vi "5-1_PushCounter.vi"() -> ()   [LabVIEW 2014]
doc: "This example demonstrates how to read one channel of digital input from a LINX device.\n------------------------------------\nAuther: Koji Ohashi\nCopyright (c) 2020 Japan LabVIEW Users Group, Volunteer members.\nThis VI is released under the MIT License.\nhttp://opensource.org/licenses/mit-license.php\n------------------------------------"
uses:
  <vilib>/MakerHub/LINX/LMH-LINX.lvlib
  <vilib>/MakerHub/LINX/Public/Peripherals/Digital/Digital Read 1 Chan.vi
  <vilib>/MakerHub/LINX/Public/Utilities/Open Serial.vi
panel:
  out "Count":i32
  out "DI Value":bool
  in  "DI Channel":u8=2
  in  "Stop Button":bool
  in  "Serial Port":refnum<visa-resource-name>
  # "LINX Device Settings"
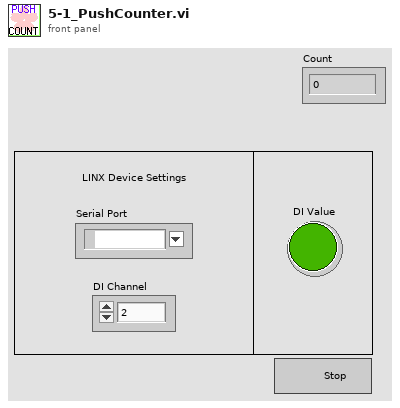
[diagram p1: front panel]
types:
  T1 = typedef "LMH-LINX.lvlib/LINX Ref.ctl" = cluster{"IO":T2, "Interface":T3, "LINX Device Config":T4}
  T2 = typedef "LMH-LINX.lvlib/Platform.ctl" = enum16{"Remote", "Local"}
  T3 = typedef "LMH-LINX.lvlib/Interface.ctl" = enum16{"Serial", "TCP"}
  T4 = typedef "LMH-LINX.lvlib/Device.lvlib/LINX Device Config.ctl" = cluster{"Interface":T3, "COM Port":refnum<visa-resource-name>, "TCP Configuration":T5, "Device Family":u8, "Device ID":u8, "Device Name":string, "TCP Ref":refnum<k5>, "Channels":T6}
  T5 = typedef "LMH-LINX.lvlib/Device.lvlib/TCP Config.ctl" = cluster{"IP Address":string, "Port":u16}
  T6 = typedef "LMH-LINX.lvlib/Channels.ctl" = cluster{"DI":u8[], "DO":u8[], "AI":u8[], "AO":u8[], "PWM":u8[], "QE":u8[], "UART":u8[], "I2C 2":u8[], "SPI":u8[], "CAN":u8[], "Servo":u8[], "AI Ref (V)":dbl, "AI Resolution (Bits)":u8, "AO Ref (V)":dbl, "AO Resolution (Bits)":u8}
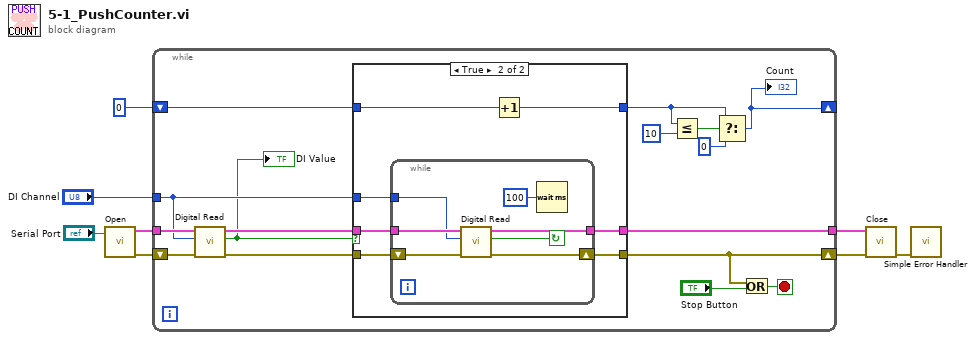
[diagram p0: block diagram]
diagram:
  n1 = call-poly <vilib>:"Open.vi"("Serial Port"="Serial Port") -> ("Error Out"=w7:errorcluster, "LINX Resource"=w8:T1)  [unwired: 8 in, 1 out]
  n2 = while {
    tunnel: w8 -> [w22]
    tunnel: [w10] -> w6
    shift-right: [w13] -> w5
    shift-left: w7 -> [w21]
    tunnel: "DI Channel" -> [w15]
    shift-right: [w17] -> _
    shift-left: 0 -> [w12]
    stop <- w24 stop-if-true
    n3 = call-poly <vilib>:"Digital Read.vi"("Error In"=w21, "DI Channel"=w15, "LINX Resource"=w22) -> ("Error Out"=w14:errorcluster, "DI Value"=w9:bool, "LINX Resource"=w16:T1)  [unwired: 6 in]
    "DI Value" <- w9
    n4 = case shown="TRUE" w9 {
      tunnel: w16 -> [w25 w34]
      tunnel: w15 -> [_ w33]
      tunnel: w14 -> [w27 w32]
      tunnel: [w27 w31] -> w13
      tunnel: w12 -> [w26 w28]
      tunnel: [w26 w30] -> w11
      tunnel: [w25 w29] -> w10
      frame False {
      }
      frame True {
        n5 = while {
          tunnel: w34 -> [w41]
          tunnel: w33 -> [w40]
          shift-right: [w38] -> w31
          shift-left: w32 -> [w39]
          tunnel: [w35] -> w29
          stop <- w36 continue-if-true
          n6 = call-poly <vilib>:"Digital Read.vi"("Error In"=w39, "DI Channel"=w40, "LINX Resource"=w41) -> ("Error Out"=w38:errorcluster, "DI Value"=w36:bool, "LINX Resource"=w35:T1)  [unwired: 6 in]
          n7 = Wait (ms)(milliseconds to wait=u32 100) -> ()  [unwired: 1 out]
        }
        n8 = Increment(x=w28) -> (x+1=w30:i32)
      }
    }
    n9 = Less Or Equal?(x=w11, y=10) -> (x <= y?=w19:bool)
    n10 = Select(t=w11, s=w19, f=0) -> (s? t:f=w17:i32)
    "Count" <- w17
    n11 = Or(x=w13, y="Stop Button") -> (x .or. y?=w24:bool)
  }
  n12 = call <vilib>:"Close.vi"("Error In"=w5, "LINX Resource"=w6) -> ("Error Out"=w3:errorcluster)  [unwired: 9 in]
  n13 = call <vilib>:"Simple Error Handler.vi"("error in (no error)"=w3) -> ()  [unwired: 4 in, 5 out]
